vi "Insert For Loop.vi"(8 "error in (no error)":errorcluster, 10 "Insert For Loop":T1, 11 "Test Executive Builder Model in":refnum<class "Test Executive Builder Model.lvclass">) -> (0 "error out":errorcluster, 3 "Test Executive Builder Model out":refnum<class "Test Executive Builder Model.lvclass">, 5 "Unique ID out":string)   [LabVIEW 2017, in "Test Executive Builder Model.lvclass"]
uses:
  Test Executive Builder Model.lvclass
  <vilib>/gpm_packages/@cs/test-executive/Source/Test Executive/TestExecutive Ref/TestExecutive Ref.lvclass
  Test Executive Builder Model Messages/Redraw Tree Msg/Redraw Tree Msg.lvclass
  <vilib>/ActorFramework/Actor/Actor.lvclass
  C:/Program Files (x86)/National Instruments/LabVIEW 2017/vi.lib/ActorFramework/Actor/Actor.lvclass
  Application Dependencies/Insert For Loop.ctl
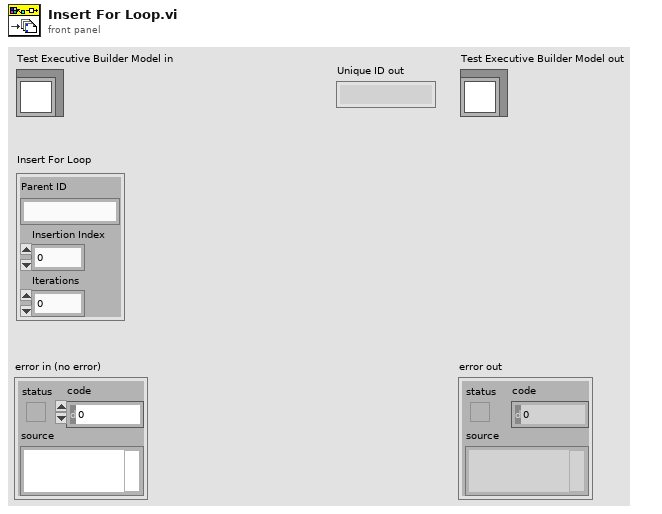
[diagram p1: front panel]
types:
  T1 = typedef "Insert For Loop.ctl" = cluster{"Parent ID":string, "Insertion Index":i32, "Iterations":i32}
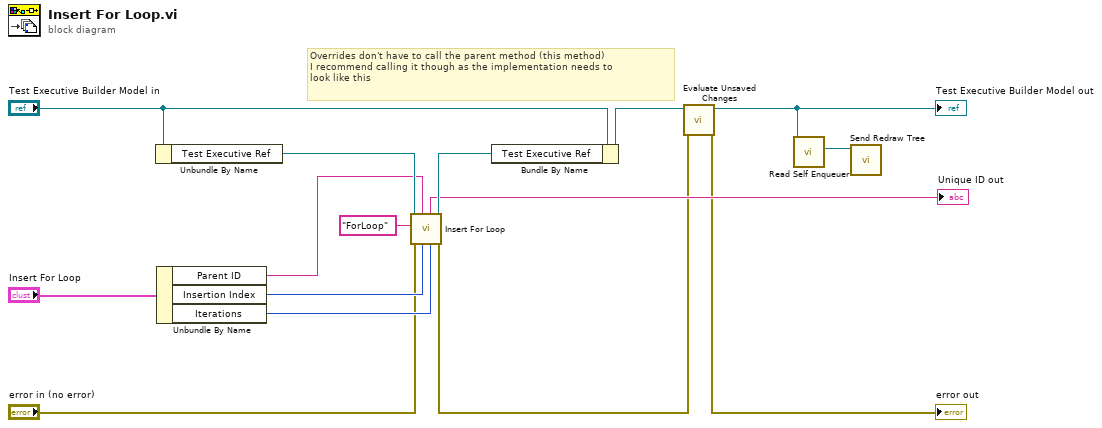
[diagram p0: block diagram]
diagram:
  # "Overrides don't have to call the parent method (this method)\nI recommend calling it though as the implementation needs to\nlook like this"
  n1 = Unbundle By Name("Test Executive Builder Model in") -> ("Test Executive Ref"=w15:refnum<data-value>)
  n2 = Unbundle By Name("Insert For Loop") -> ("Parent ID"=w13:string, "Insertion Index"=w12:i32, "Iterations"=w11:i32)
  n3 = call <vilib>:"Insert For Loop.vi"("Loop Iterations"=w11, "Insertion Index"=w12, "Parent ID"=w13, "error in (no error)"="error in (no error)", "Name"="ForLoop", "Test Executive Ref"=w15) -> ("error out"=w2:errorcluster, "Test Executive Ref out"=w9:refnum<data-value>, "Unique ID out"=→"Unique ID out":string)  [unwired: 2 in, 1 out]
  n4 = Bundle By Name(cluster="Test Executive Builder Model in", "Test Executive Ref"=w9) -> (w4:refnum<class "Test Executive Builder Model.lvclass">)
  n5 = call-dynamic "Evaluate Unsaved Changes.vi"("error in (no error)"=w2, "Test Executive Builder Model in"=w4) -> ("error out"=→"error out":errorcluster, "Test Executive Builder Model out"=w3:refnum<class "Test Executive Builder Model.lvclass">)  [unwired: 8 in]
  "Test Executive Builder Model out" <- w3
  n6 = call <vilib>:"Read Self Enqueuer.vi"("Actor"=w3) -> ("Self Enqueuer"=w6:refnum<class "Message Enqueuer.lvclass">)  [unwired: 10 in]
  n7 = call "Send Redraw Tree.vi"("Message Enqueuer"=w6) -> ()  [unwired: 9 in, 2 out]
